vi "Find_Unmoving_Dots_for_Gap_Closing-2.vi"(6 "Gaps for closing":i32, 7 "dR min":dbl, 8 "i+j":i32, 9 "Y":dbl, 10 "X":dbl, 11 "(X,Y) IN":dbl[][](array[numeric])) -> (0 "Count of \ngaps between\ndots":i32, 1 "Y OUT":dbl, 2 "X OUT":dbl, 3 "Gap Potentially \nClosed":bool, 4 "Index of \ncandidate dot\ninside the frame":i32)   [LabVIEW 2013]
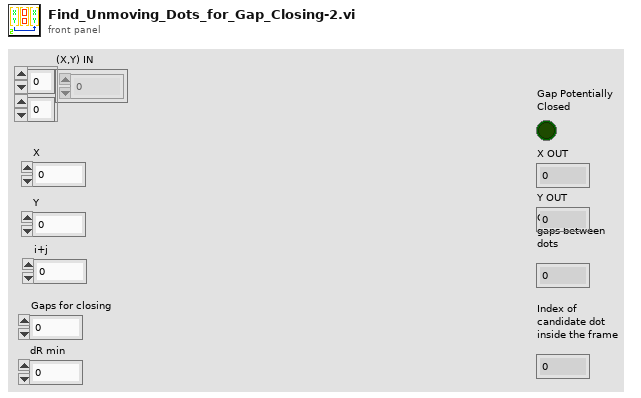
[diagram p1: front panel]
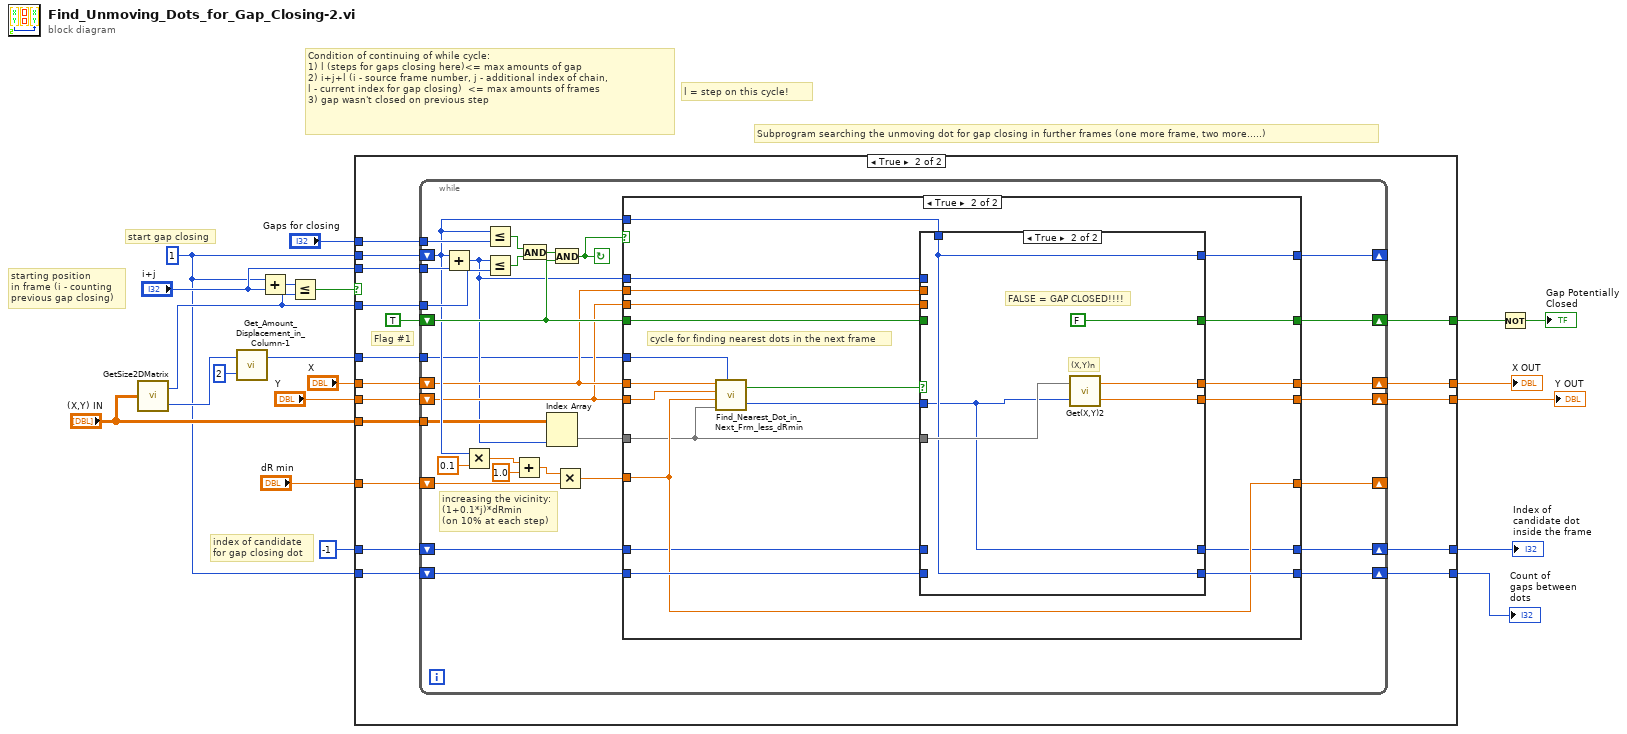
[diagram p0: block diagram]
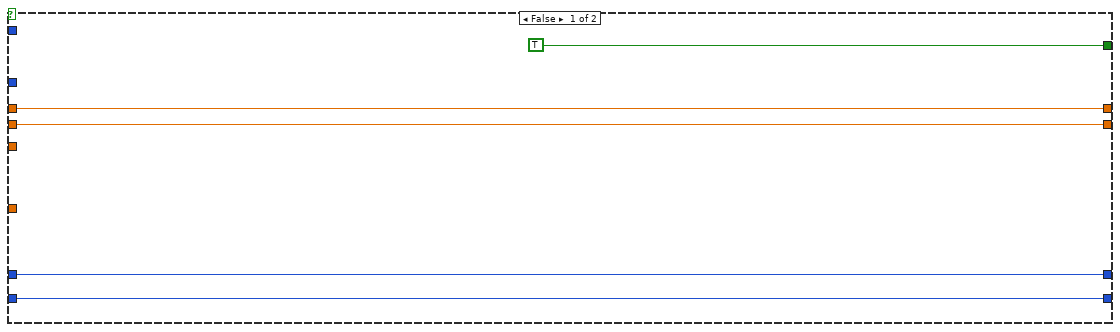
[diagram p2: hidden frame]
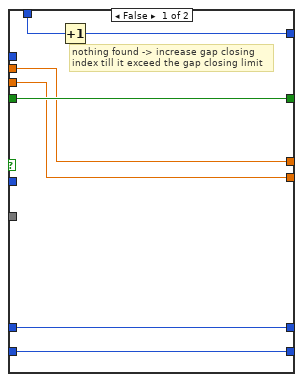
[diagram p4: hidden frame]
diagram:
  w3 = 1
  # "index of candidate \nfor gap closing dot"
  # "starting position\nin frame (i - counting\nprevious gap closing)"
  # "start gap closing"
  # "Subprogram searching the unmoving dot for gap closing in further frames (one more frame, two more.....)"
  # "l = step on this cycle!"
  # "Condition of continuing of while cycle:\n1) l (steps for gaps closing here)<= max amounts of gap\n2) i+j+l (i - source frame number, j - additional index of chain, \nl - current index for gap closing)  <= max amounts of frames\n3) gap wasn't closed on previous step"
  n1 = call "GetSize2DMatrix.vi"("Array IN (2D)"="(X,Y) IN") -> ("# Cols"=w5:i32, "# Rows"=w8:i32)
  n2 = call "Get_Amount_Displacement_in_Column-1.vi"("multiplier"=2 ("y"), "# Rows"=w8) -> ("Displ amount"=w4:i32)  [unwired: 1 out]
  n3 = Add(x=w3, y="i+j") -> (x+y=w19:i32)
  n4 = Less Or Equal?(x=w19, y=w5) -> (x <= y?=w20:bool)
  n5 = case shown="True" w20 {
    tunnel: w3 -> [_ w42]
    tunnel: w5 -> [_ w41]
    tunnel: w3 -> [w25 w32]
    tunnel: [w25 w31] -> w13
    tunnel: "i+j" -> [_ w40]
    tunnel: "(X,Y) IN" -> [_ w39]
    tunnel: "Gaps for closing" -> [_ w38]
    tunnel: "X" -> [w23 w36]
    tunnel: "Y" -> [w22 w35]
    tunnel: "dR min" -> [_ w34]
    tunnel: [TRUE w33] -> w12
    tunnel: [w23 w30] -> w10
    tunnel: [w22 w29] -> w9
    tunnel: w4 -> [_ w28]
    tunnel: -1 -> [w21 w27]
    tunnel: [w21 w26] -> w1
    frame False {
    }
    frame True {
      # "Flag #1"
      n6 = while {
        shift-right: [w53] -> _
        shift-left: w42 -> [w60]
        tunnel: w41 -> [w71]
        tunnel: w40 -> [w72]
        tunnel: w38 -> [w70]
        shift-right: [w56] -> w33
        shift-left: TRUE -> [w65]
        shift-right: [w54] -> w31
        shift-left: w32 -> [w55]
        shift-right: [w52] -> w30
        shift-left: w36 -> [w50]
        shift-right: [w51] -> w29
        shift-left: w35 -> [w49]
        shift-right: [w46] -> _
        shift-left: w34 -> [w62]
        tunnel: w28 -> [w45]
        tunnel: w39 -> [w48]
        shift-right: [w43] -> w26
        shift-left: w27 -> [w44]
        stop <- w66 continue-if-true
        # "increasing the vicinity:\n(1+0.1*j)*dRmin\n(on 10% at each step)"
        n7 = Add(x=w60, y=w72) -> (x+y=w47:i32)
        n8 = Multiply(x=w60, y=0.1) -> (x*y=w58:dbl)
        n9 = Less Or Equal?(x=w60, y=w70) -> (x <= y?=w69:bool)
        n10 = Less Or Equal?(x=w47, y=w71) -> (x <= y?=w68:bool)
        n11 = Add(x=w58, y=1.0 ("x")) -> (x+y=w57:dbl)
        n12 = And(x=w69, y=w68) -> (x .and. y?=w67:bool)
        n13 = Index Array(array=w48, index (col)=w47) -> (element=w64:dbl[])  [unwired: 1 in]
        n14 = And(x=w67, y=w65) -> (x .and. y?=w66:bool)
        n15 = Multiply(x=w57, y=w62) -> (x*y=w63:dbl)
        n16 = case shown="True" w66 {
          tunnel: w60 -> [w77 w96]
          tunnel: w65 -> [w78 w99]
          tunnel: w50 -> [w76 w87]
          tunnel: w49 -> [w75 w86]
          tunnel: w64 -> [_ w82]
          tunnel: w63 -> [w74 w85]
          tunnel: [w78 w98] -> w56
          tunnel: w55 -> [w79 w97]
          tunnel: [w79 w95] -> w54
          tunnel: [w77 w94] -> w53
          tunnel: [w76 w93] -> w52
          tunnel: [w75 w92] -> w51
          tunnel: w50 -> [_ w91]
          tunnel: w49 -> [_ w90]
          tunnel: w47 -> [_ w89]
          tunnel: [w74 w85] -> w46
          tunnel: w45 -> [_ w88]
          tunnel: w44 -> [w73 w81]
          tunnel: [w73 w80] -> w43
          frame False {
          }
          frame True {
            # "cycle for finding nearest dots in the next frame"
            n17 = call "Find_Nearest_Dot_in_Next_Frm_less_dRmin.vi"("X"=w87, "Y"=w86, "dR min"=w85, "n+1 frame\ncolumn (X,Y)"=w82, "Max number\nof dots in \ncolumn (X,Y)"=w88) -> ("Any dots found?"=w84:bool, "index of the dot \nwith minimal displ"=w83:i32)
            n18 = case shown="True" w84 {
              tunnel: w99 -> [w105 _]
              tunnel: [w105 FALSE] -> w98
              tunnel: w82 -> [_ w111]
              tunnel: w97 -> [w106 _]
              tunnel: w96 -> [w104 w108]
              tunnel: [w106 w108] -> w95
              tunnel: [w103 w108] -> w94
              tunnel: [w102 w110] -> w93
              tunnel: [w101 w109] -> w92
              tunnel: w91 -> [w102 _]
              tunnel: w90 -> [w101 _]
              tunnel: w89 -> [_ _]
              tunnel: w83 -> [_ w107]
              tunnel: w81 -> [w100 _]
              tunnel: [w100 w107] -> w80
              frame False {
                # "nothing found -> increase gap closing\nindex till it exceed the gap closing limit"
                n19 = Increment(x=w104) -> (x+1=w103:i32)
              }
              frame True {
                # "(X,Y)n"
                # "FALSE = GAP CLOSED!!!!"
                n20 = call "Get(X,Y)2.vi"("[IN] index of (X,Y)"=w107, "[IN] Array coordi\nnates (X,Y) in Frame"=w111) -> ("[OUT] Y"=w109:dbl, "[OUT] X"=w110:dbl)
              }
            }
          }
        }
      }
    }
  }
  "Count of \ngaps between\ndots" <- w13
  "X OUT" <- w10
  "Y OUT" <- w9
  "Index of \ncandidate dot\ninside the frame" <- w1
  n21 = Not(x=w12) -> (.not. x?=→"Gap Potentially \nClosed":bool)
